vi "VerifyArguments.vi"(8 "error in (no error)":errorcluster, 11 "RunVI in":refnum<class "RunVI.lvclass">) -> (0 "error out":errorcluster, 3 "RunVI out":refnum<class "RunVI.lvclass">)   [LabVIEW 2014, in "RunVI.lvclass"]
uses:
  RunVI.lvclass
  RunVI.lvclass/RunVI.ctl
  Utilities/OperationErrorType.ctl
panel:
  in  "Error message":string="-VIPath cannot be empty."
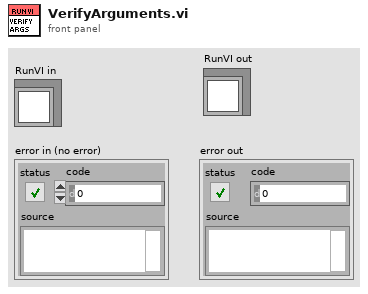
[diagram p1: front panel]
types:
  T1 = typedef "OperationErrorType.ctl" = enum16{"RequiredArgumentMissing", "UnknownArguments", "LoggerSetMultipleTimes", "OperationBrokenError"}
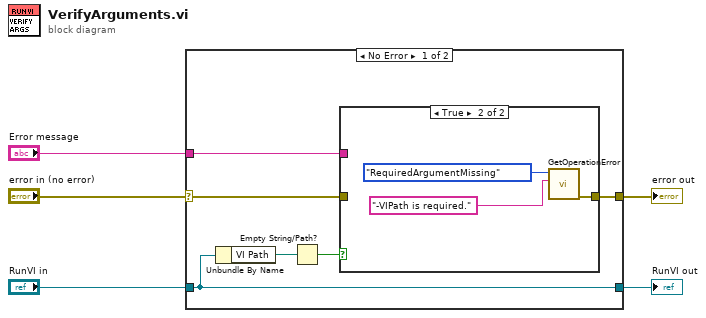
[diagram p0: block diagram]
diagram:
  n1 = case shown="No Error" "error in (no error)" {
    selector: "error in (no error)" -> [w8 w16]
    tunnel: [w10 w16] -> w5
    tunnel: "RunVI in" -> [w7 w17]
    tunnel: [w7 w17] -> w2
    tunnel: "Error message" -> [w6 _]
    frame No Error {
      n2 = Unbundle By Name(w7) -> ("VI Path"=w11:path)
      n3 = Empty String/Path?(string/path=w11) -> (empty?=w9:bool)
      n4 = case shown="True" w9 {
        tunnel: w8 -> [w12 _]
        tunnel: [w12 w15] -> w10
        tunnel: w6 -> [_ _]
        frame False {
        }
        frame True {
          n5 = call "GetOperationError.vi"("Additional Information"="-VIPath is required.", "Operation Error Type"=OperationErrorType."RequiredArgumentMissing") -> ("error out"=w15:errorcluster)  [unwired: 9 in]
        }
      }
    }
    frame Error {
    }
  }
  "error out" <- w5
  "RunVI out" <- w2
